vi "PC Streaming Host.vi"() -> ()   [LabVIEW 2012]
uses:
  <vilib>/userdefined/High Color/nirio_resource_hc.ctl
  <vilib>/FPGAPlugInAG/PXI-7951R/niLvFpga_Open_PXI-7951R.vi
  <vilib>/rvi/interface/common/dynamic/niFpgaDynamicAddResources.vi
  <vilib>/Utility/error.llb/Error Cluster From Error Code.vi
  <vilib>/LabVIEW Targets/FPGA/FlexRIO/CustomFPGAMethods/79XXR_Method_IOModuleStatusImpl.vi
  <vilib>/FPGAPlugInAG/Dynamic/niLvFpga_Run_Dynamic.vi
  <vilib>/rvi/errors/niLvFpgaAdjustHostInterfaceError.vi
  <vilib>/FPGAPlugInAG/Dynamic/niLvFpga_Close_Dynamic.vi
  <vilib>/rvi/interface/nirviOpenFPGA/nirviOpenFPGA.xnode
  FPGA Bitfiles/TopLevelFPGA2.0.lvbitx
  <vilib>/rvi/interface/nirviMethod/nirviMethod.xnode
  <vilib>/rvi/interface/nirviReadWriteControl/nirviReadWriteControl.xnode
  <vilib>/rvi/interface/nirviCloseFPGA/nirviCloseFPGA.xnode
  <vilib>/rvi/errors/niLvFpgaMergeErrorWithErrorCode.vi
  <vilib>/ptbypt/NI_PtbyPt.lvlib
  <vilib>/rvi/interface/Simulation/niFpgaSimulationCallBeginRW.vi
  RT_binary.vi
  NiFpgaLv.dll
  <vilib>/FPGAPlugInAG/Dynamic/niLvFpga_ConfigureFifo_Dynamic.vi
  <vilib>/FPGAPlugInAG/Dynamic/niLvFpga_StartFifo_Dynamic.vi
  <vilib>/FPGAPlugInAG/Dynamic/niLvFpga_ReadFifo_Dynamic.vi
panel:
  out "created path":path
  out "File name":string
  out "Total Data Chunks to Write":dbl
  in  "Tab Control":T1(tab)
  in  "Write mode":bool
  out "directory exists - please wait":u8(slide)
  out "directory ok":bool
  in  "Write Enable":bool
  in  "File Path":path=path "D:/Users/reuterc/Desktop"
  in  "Number of Files to Write":u32=1
  in  "Save 10% of Data?":bool
  out "File Writing Progress (%)":dbl(slide) scale=0.0..100.0
  in  "Location":i16(ring) items=["Purdue", "NIKHEF", "Zurich", "???"]
  in  "PXI address":T2 caption="RIO Device"
  in  "Trigger level":i16[](array[numeric])=[4000, 4000, 4000, 4000, 4000, 4000, 4000, 4000] caption="Trigger"
  in  "Channel 0":bool caption="Channel 1"
  in  "Channel 1":bool
  in  "Channel 2":bool caption="Channel 1"
  in  "Channel 3":bool caption="Channel 1"
  in  "Channel 4":bool caption="Channel 1"
  in  "Channel 5":bool caption="Channel 1"
  in  "Channel 6":bool caption="Channel 1"
  in  "Channel 7":bool caption="Channel 1"
  in  "Sources":string[](array[combo])
  in  "Serial numbers":string[](array[combo])
  in  "voltage":string[](array[string])
  in  "det_type":string[](array[combo])
  in  "Master Pulser On/Off":bool
  in  "Pulse duration (samples)":u32
  in  "Pulse Separation (samples)":u32
  in  "Testpulse Turnaround Time (samples)":u32=14
  in  "circular buffer length (samples)":u32=1000
  in  "Pretrigger Samples":u32=15
  out "Samples per Data Chunk":u32
  in  "Waveforms per Data Chunk":u32=5000 format="%.2p"
  in  "Samples per Waveform":u32=95
  in  "Data Chunks per File":u32=1000
  out "Average Throughput":dbl(graph)
  out "Loop Time":u32
  out "Inst. Throughput":dbl format="%#_6p"
  out "Elements in FIFO":u32(graph)
  out "FIFO Overflow":bool
  out "Current Chunk":u32
  out "Current File":i32
  out "Trigger rate":dbl(graph)
  out "Waveform Graph":dynamicdata(graph)
  out "Channel number displayed":i16=-1
  out "XML String":string
  out "error out":errorcluster
  out "UTC format?":bool=TRUE
  out "Stopped":bool
  out "Channel On/Off":bool[](array[boolean])
  in  "stop 2":bool
  in  "stop":bool
  # "Only write every 10th chunk to disk"
  # "Program will stop when number of Files to Write is Complete OR if stop is pressed."
  # "Write continuously"
  # "Write finite number of files"
  # "TODO: Make this look like the \"detectors\" tab"
  # "Waveform/Data Chunk information"
  # "To compare directly on a scope: Horizontal scale: 200 ns/div Vertical scale: ~100 mV/div If 15 pretriggers, delay = 700 ns"
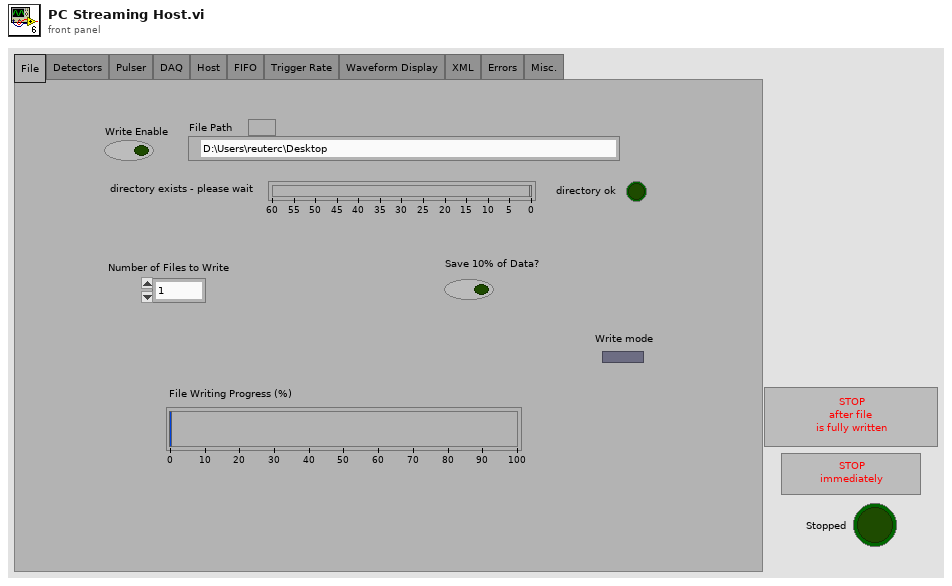
[diagram p1: front panel]
types:
  T1 = enum32{"File", "Detectors", "Pulser", "DAQ", "Host", "FIFO", "Trigger Rate", "Waveform Display", "XML", "Errors", "Misc."}
  T2 = typedef "nirio_resource_hc.ctl" = tag
  T3 = enum16{"open", "replace", "create", "open or create", "replace or create", "replace or create with confirmation"}
  T4 = enum16{"big-endian, network order", "native, host order", "little-endian"}
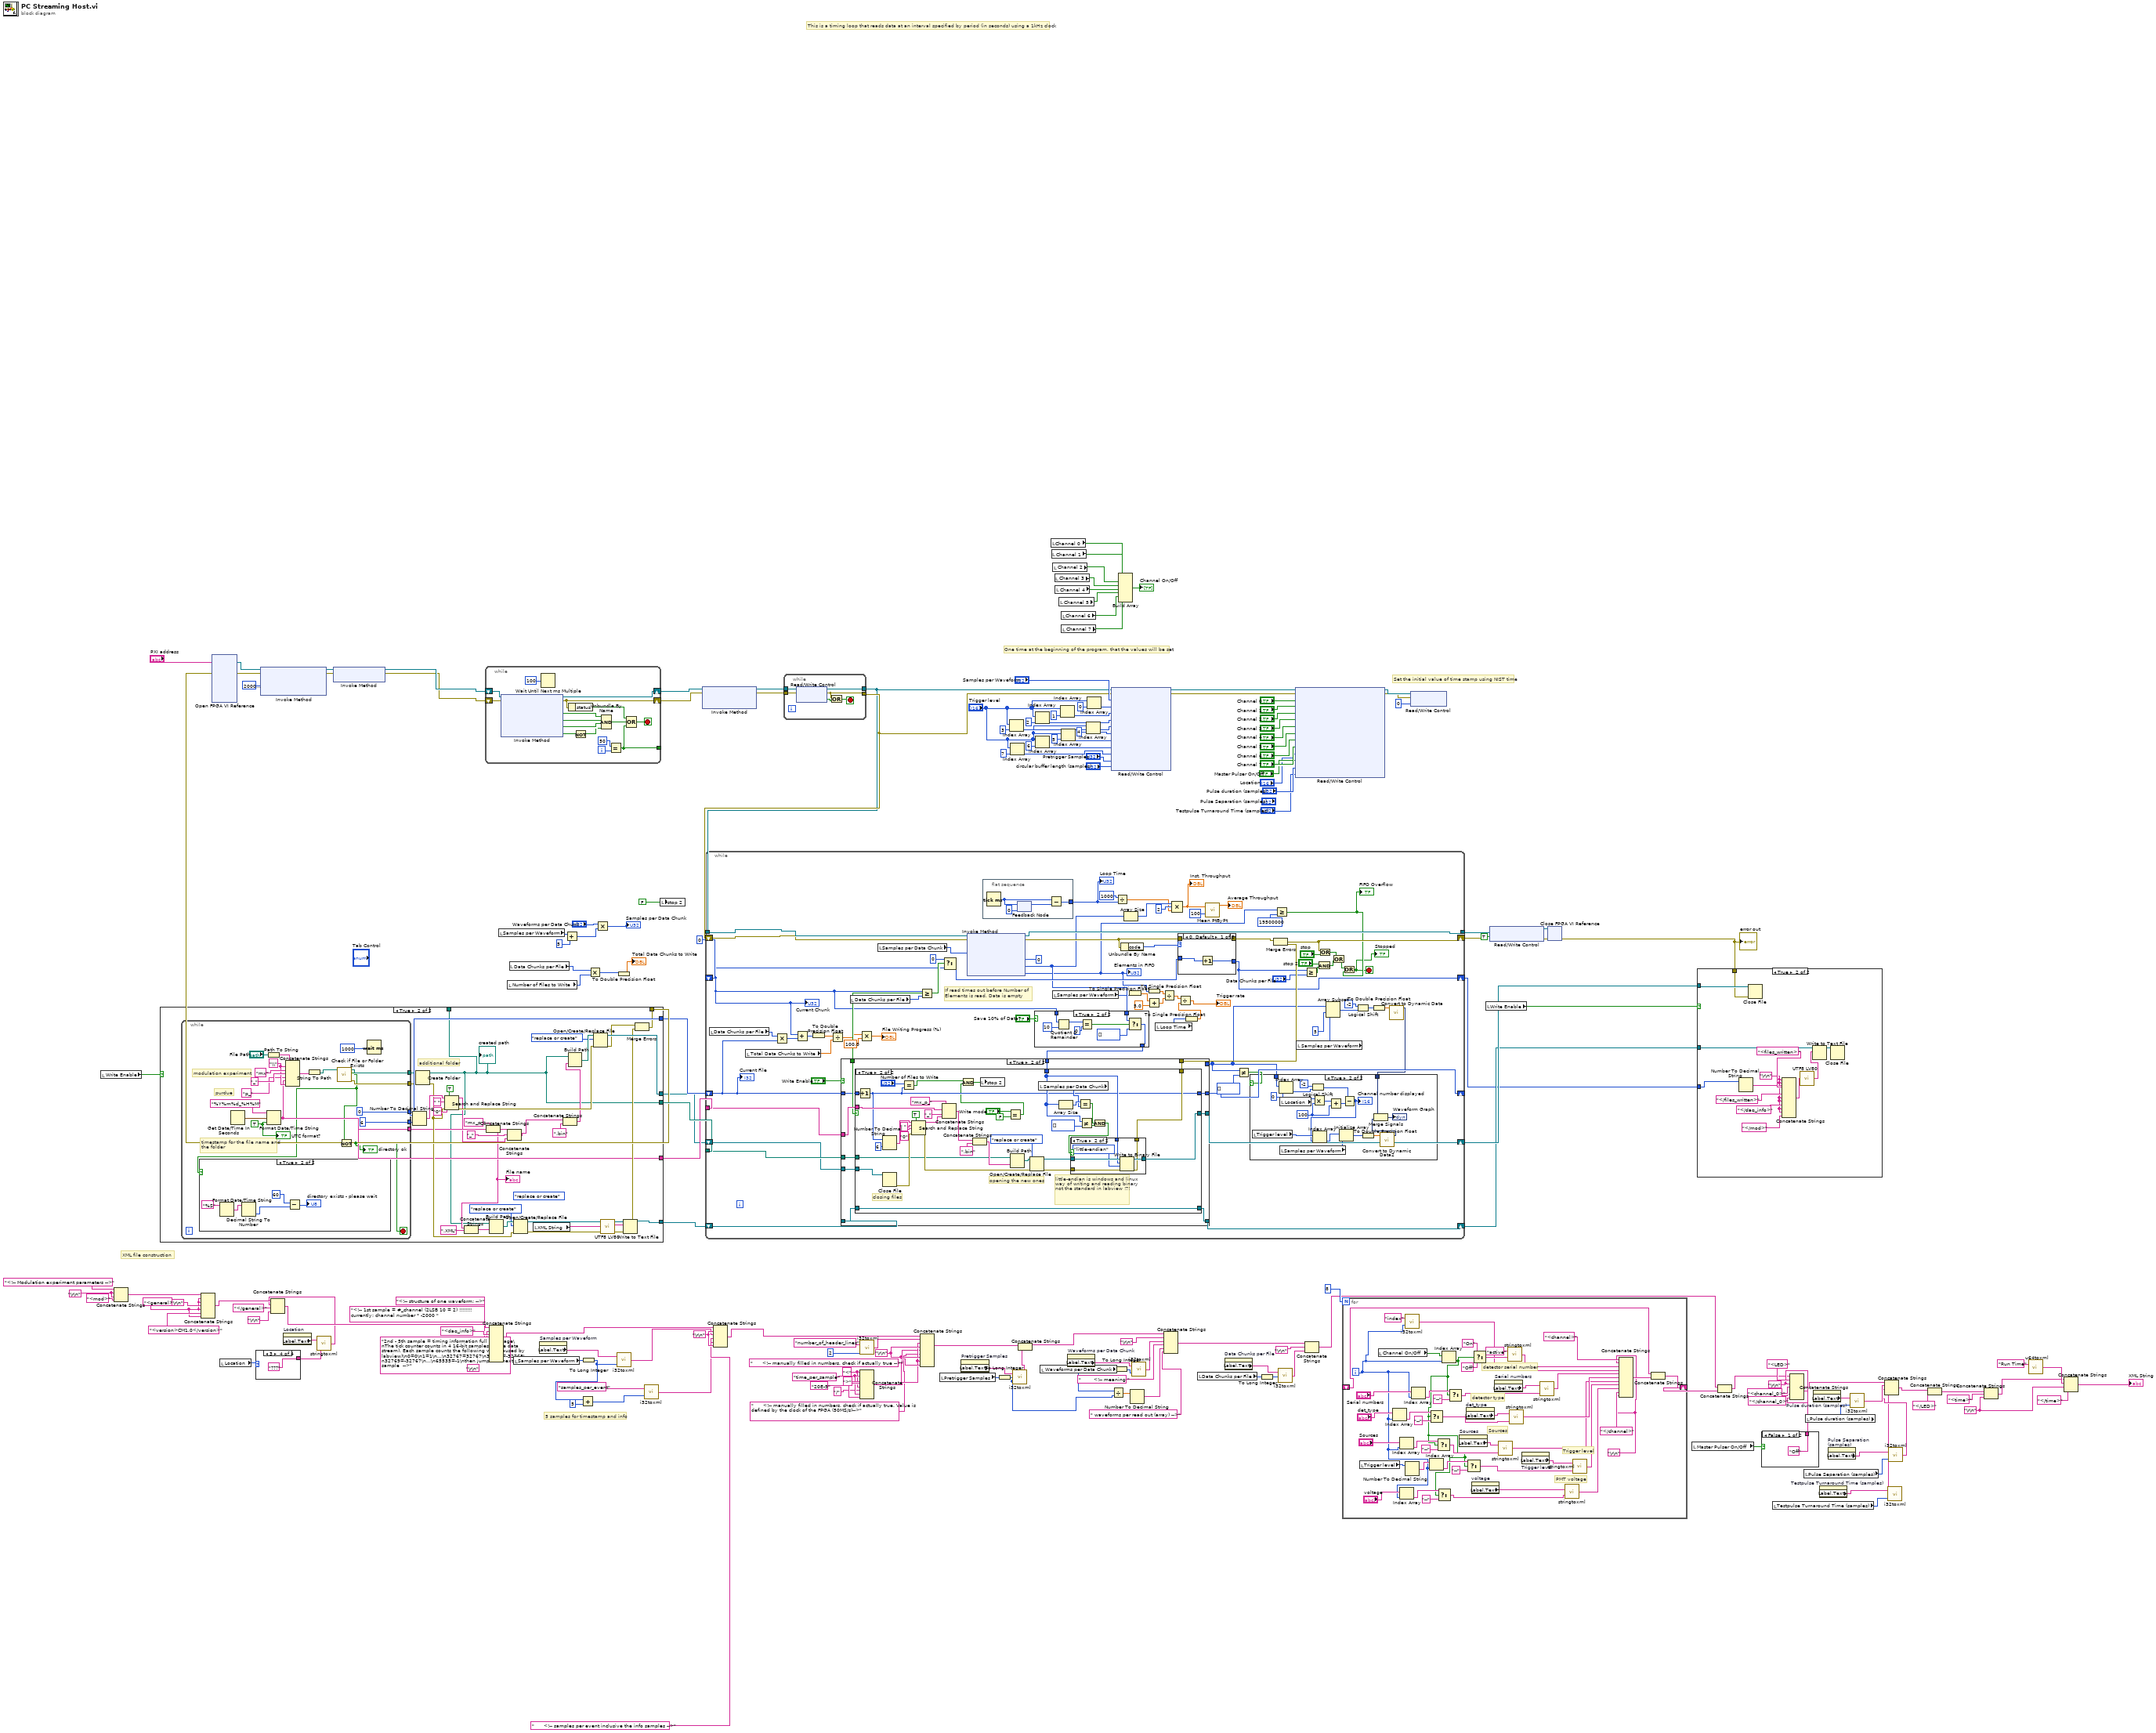
[diagram p0: block diagram]
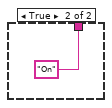
[diagram p2: hidden frame]
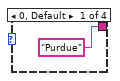
[diagram p3: hidden frame]
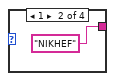
[diagram p4: hidden frame]
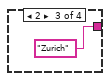
[diagram p5: hidden frame]
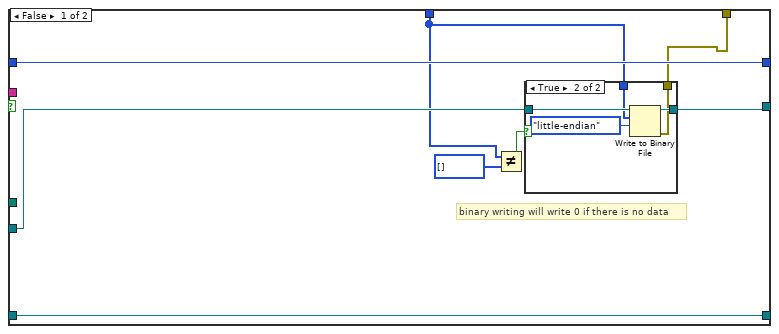
[diagram p12: hidden frame]
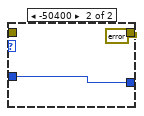
[diagram p15: hidden frame]
diagram:
  w20 = "\r\n"
  w53 = "\r\n"
  w102 = ">" ("string")
  w99 = "<" ("string")
  w101 = "time_per_sample" ("variable name")
  w106 = "      <!-- manually filled in numbers, check if actually true -->" ("string")
  w107 = "\r\n"
  w116 = "\r\n"
  w61 = "\r\n"
  w69 = "\r\n"
  w133 = "\r\n"
  # "This is a timing loop that reads data at an interval specified by period (in seconds) using a 1kHz clock"
  # "Set the initial value of time stamp using NIST time"
  # "5 samples for timestamp and info"
  # "XML file construction"
  # "One time at the beginning of the program, that the values will be set"
  n1 = local read "Write Enable"() -> (w170:bool)
  n2 = Concatenate Strings("<!-- Modulation experiment parameters -->", w133, w133, "<mod>" ("string")) -> (w73:string)
  n3 = case shown="True" w170 {
    tunnel: [_ w184] -> w175
    tunnel: [_ w193] -> w174
    tunnel: [_ w205] -> w173
    tunnel: [_ w211] -> w171
    tunnel: [_ w207] -> w169
    tunnel: [_ w194] -> w167
    tunnel: [_ w184] -> _
    frame False {
    }
    frame True {
      (unwired) T3."replace or create" ("operation (0:open)")
      # "additional folder"
      n4 = while {
        tunnel: [i16 6 ("width (-)")] -> w216
        tunnel: [0 ("number")] -> w211
        tunnel: [w225] -> w193
        tunnel: [w222] -> w187
        tunnel: [w221] -> w186
        stop <- w218 stop-if-true
        w226 = "\\" ("string")
        w230 = TRUE ("UTC format")
        # "modulation experiment"
        # "purdue"
        # "timestamp for the file name and the folder"
        n5 = Get Date/Time In Seconds() -> (seconds since 1Jan1904=w231:timestamp)
        n6 = Path To String(path="File Path") -> (string=w233:string)
        n7 = Format Date/Time String(time format string (%c)="%Y%m%d_%H%M", seconds (now)=w231, UTC format=w230) -> (date/time string=w225:string)
        n8 = Concatenate Strings(w233, w226, "mx" ("string"), "_" ("string"), "p_" ("string"), w225, w226) -> (w236:string)
        n9 = String To Path(string=w236) -> (path=w223:path)
        n10 = call <vilib>:"Check if File or Folder Exists.vi"("path"=w223) -> ("error out"=w222:errorcluster, "file or folder exists?"=w220:bool, "dup path"=w221:path)  [unwired: 8 in]
        n11 = case shown="True" w220 {
          frame False {
          }
          frame True {
            n12 = Format Date/Time String(time format string (%c)="%S") -> (date/time string=w240:string)  [unwired: 2 in]
            n13 = Decimal String To Number(string=w240) -> (number=w238:i32)  [unwired: 2 in, 1 out]
            n14 = Subtract(x=60, y=w238) -> (x-y=→"directory exists - please wait":i32)
          }
        }
        n15 = Not(x=w220) -> (.not. x?=w218:bool)
        "directory ok" <- w218
        n16 = Wait (ms)(milliseconds to wait=1000) -> ()  [unwired: 1 out]
        "UTC format?" <- w230
      }
      n17 = Number To Decimal String(number=w211, width (-)=w216) -> (decimal integer string=w215:string)
      n18 = Create Folder(path (use dialog)=w186, error in=w187) -> (created path=w184:path, error out=w202:errorcluster)  [unwired: 1 in, 1 out]
      "created path" <- w184
      n19 = Search and Replace String(replace all?=TRUE ("replace all? (F)"), input string=w215, search string=" ", replace string="0" ("replace string (\"\")"), error in=w202) -> (result string=w192:string, error out=w209:errorcluster)  [unwired: 3 in, 2 out]
      n20 = Concatenate Strings("mx_p_" ("string"), w193) -> (w185:string)
      "File name" <- w185
      n21 = Concatenate Strings(w185, ".XML" ("substring (\"\")")) -> (w199:string)
      n22 = Build Path(base path=w184, name or relative path=w199) -> (appended path=w204:path)
      n23 = Concatenate Strings(w185, "_" ("string"), w192) -> (w188:string)
      n24 = Open/Create/Replace File(file path (use dialog)=w204, error in=w202, operation (0:open)=T3."replace or create") -> (refnum out=w195:refnum<file>, error out=w197:errorcluster)  [unwired: 3 in, 1 out]
      n25 = local read "XML String"() -> (w189:string)
      n26 = Concatenate Strings(w188, ".bin" ("substring (\"\")")) -> (w201:string)
      n27 = Build Path(base path=w184, name or relative path=w201) -> (appended path=w210:path)
      n28 = Open/Create/Replace File(file path (use dialog)=w210, error in=w209, operation (0:open)=T3."replace or create") -> (refnum out=w207:refnum<file>, error out=w206:errorcluster)  [unwired: 3 in, 1 out]
      n29 = call "UTF8 LV80.vi"("text"=w189) -> ("utf-8 text out"=w190:string)
      n30 = Write to Text File(file (use dialog)=w195, text=w190, error in=w197) -> (refnum out=w194:refnum<file>, error out=w196:errorcluster)  [unwired: 1 in, 1 out]
      n31 = Merge Errors(w206, w196) -> (w205:errorcluster)
    }
  }
  n32 = Concatenate Strings(w73, w69, w69, "<general>" ("string"), w69, "<version>CM1.0</version>" ("string"), w69) -> (w74:string)
  n33 = xnode "Open FPGA VI Reference"("error in"=w173, "resource name"="PXI address") -> ("FPGA VI Reference Out"=w183:refnum<k20>, "error out"=w182:errorcluster)
  n34 = local read "Location"() -> (w71:i16)
  n35 = case shown="3" w71 {
    tunnel: ["Purdue" "NIKHEF" "Zurich" "???"] -> w70
    frame 0, Default {
    }
    frame 1 {
    }
    frame 2 {
    }
    frame 3 {
    }
  }
  n36 = xnode "Invoke Method"("FPGA VI Reference In"=w183, "error in"=w182, "Requested Depth"=u32 20000000) -> ("FPGA VI Reference Out"=w60:refnum<k20>, "error out"=w59:errorcluster)  [unwired: 1 out]
  n37 = property on="Location" class="Ring (strict)"() -> ("Label.Text"=w38:string)  [unwired: 2 in, 2 out]
  n38 = call "stringtoxml.vi"("String to write"=w70, "XML Tag"=w38) -> ("xml string"=w68:string)
  n39 = Concatenate Strings(w74, w68, "</general>" ("string"), "\r\n") -> (w75:string)
  n40 = xnode "Invoke Method"("FPGA VI Reference In"=w60, "error in"=w59) -> ("FPGA VI Reference Out"=w3:refnum<k20>, "error out"=w2:errorcluster)
  n41 = while {
    shift-right: [w252] -> w179
    shift-left: w2 -> [w260]
    shift-right: [w259] -> w12
    shift-left: w3 -> [w261]
    tunnel: [w248] -> _
    i -> [w254]
    stop <- w249 stop-if-true
    n42 = xnode "Invoke Method"("FPGA VI Reference In"=w261, "error in"=w260) -> ("FPGA VI Reference Out"=w259:refnum<k20>, "error out"=w252:errorcluster, "IO Module Present?"=w258:bool, "Power Enabled?"=w257:bool, "IO Enabled?"=w256:bool, "IO Module Mismatch?"=w247:bool)
    n43 = Wait Until Next ms Multiple(millisecond multiple=u32 100) -> ()  [unwired: 1 out]
    n44 = Unbundle By Name(w252) -> ("status"=w251:bool)
    n45 = Not(x=w247) -> (.not. x?=w246:bool)
    n46 = Compound Arithmetic op=AND(w258, w257, w256, w246) -> (w250:bool)
    n47 = Equal?(x=50, y=w254) -> (x = y?=w248:bool)
    n48 = Compound Arithmetic op=OR(w251, w250, w248) -> (w249:bool)
  }
  n49 = Concatenate Strings(w75, w61, "<daq_info>" ("string"), w61, "<!-- structure of one waveform: -->", w61, "<!-- 1st sample = #_channel (2LSB 10 = 2) !!!!!!!! currently: channel number * -2000 " ("string"), w61, "2nd - 5th sample = timing information full I16 usage\nThe tick counter counts in 4 16-bit samples (in the data stream). Each sample counts the following way (caused by labview)\n0=0\n1=1\n…\n32767=32767\n32768=-32768\n32769=-32767\n…\n65535=-1\nthen jump into next sample  -->" ("string"), w61) -> (w76:string)
  n50 = local read "Samples per Waveform"() -> (w39:u32)
  n51 = local read "Number of Files to Write"() -> (w27:u32)
  n52 = local read "Data Chunks per File"() -> (w28:u32)
  n53 = local read "Samples per Waveform"() -> (w108:u32)
  n54 = property on="Samples per Waveform" class="DigNum (strict)"() -> ("Label.Text"=w37:string)  [unwired: 2 in, 2 out]
  n55 = Add(x=w39, y=u32 5) -> (x+y=w41:u32)
  n56 = To Long Integer(number=w108) -> (32bit integer=w111:i32)
  n57 = Add(x=w111, y=5) -> (x+y=w113:i32)
  n58 = Multiply(x=w28, y=w27) -> (x*y=w26:u32)
  n59 = Multiply(x="Waveforms per Data Chunk", y=w41) -> (x*y=→"Samples per Data Chunk":u32)
  n60 = call "i32toxml.vi"("variable"=w111, "variable name"=w37) -> ("xml string"=w109:string)
  n61 = To Double Precision Float(number=w26) -> (double precision float=→"Total Data Chunks to Write":dbl)
  n62 = call "i32toxml.vi"("variable"=w113, "variable name"="samples_per_event") -> ("xml string"=w114:string)
  n63 = local write "stop 2"(FALSE ("stop 2")) -> ()
  n64 = xnode "Invoke Method"("FPGA VI Reference In"=w12, "error in"=w179) -> ("FPGA VI Reference Out"=w180:refnum<k20>, "error out"=w181:errorcluster)  [unwired: 1 in]
  n65 = Concatenate Strings(w76, w116, w109, w114, "      <!-- samples per event inclusive the info samples -->" ("string"), w116) -> (w77:string)
  n66 = while {
    tunnel: [w262] -> w135
    tunnel: [w267] -> w11
    tunnel: w180 -> [w266]
    tunnel: w181 -> [w265]
    stop <- w263 stop-if-true
    n67 = xnode "Read/Write Control"("FPGA VI Reference In"=w266, "error in"=w265) -> ("FPGA VI Reference Out"=w267:refnum<k20>, "error out"=w262:errorcluster, "Init Done"=w264:bool)
    n68 = Or(x=w262, y=w264) -> (x .or. y?=w263:bool)
  }
  n69 = while {
    shift-right: [w322] -> w14
    shift-left: w135 -> [w283]
    tunnel: w174 -> [w328]
    shift-right: [w313] -> w136
    shift-left: u32 0 -> [w291]
    tunnel: w175 -> [w329]
    shift-right: [w324] -> _
    shift-left: w171 -> [w294]
    shift-right: [w319] -> w168
    shift-left: w169 -> [w320]
    shift-right: [w316] -> w166
    shift-left: w167 -> [w317]
    tunnel: w11 -> [w284]
    tunnel: [w341] -> w15
    stop <- w268 stop-if-true
    # "If read times out before Number of Elements is read, Data is empty"
    n70 = local read "Data Chunks per File"() -> (w293:u32)
    n71 = local read "Total Data Chunks to Write"() -> (w288:dbl)
    n72 = Multiply(x=w293, y=w294) -> (x*y=w292:u32)
    n73 = Add(x=w291, y=w292) -> (x+y=w290:u32)
    n74 = To Double Precision Float(number=w290) -> (double precision float=w289:dbl)
    n75 = Divide(x=w289, y=w288) -> (x/y=w286:dbl)
    n76 = local read "Data Chunks per File"() -> (w303:u32)
    n77 = Multiply(x=w286, y=100.0) -> (x*y=→"File Writing Progress (%)":dbl)
    n78 = local read "Samples per Data Chunk"() -> (w295:u32)
    n79 = Greater Or Equal?(x=w291, y=w303) -> (x >= y?=w325:bool)
    n80 = Select(t=u32 0, s=w325, f=w291) -> (s? t:f=w326:u32)
    n81 = xnode "Invoke Method"("FPGA VI Reference In"=w284, "error in"=w283, "Number of Elements"=w295, "Timeout (ms)"=0) -> ("FPGA VI Reference Out"=w341:refnum<k20>, "error out"=w338:errorcluster, "Data"=w300:i16[], "Elements Remaining"=w282:u32)
    "Elements in FIFO" <- w282
    n82 = flat-sequence {
      tunnel: [w372] -> w332
      frame #0 {
        n83 = Tick Count (ms)() -> (millisecond timer value=w371:u32)
        n84 = feedback #1(u32 0 ("millisecond timer value")) -> (w370:u32)
        n85 = feedback-in #1(w371) -> ()
        n86 = Subtract(x=w371, y=w370) -> (x-y=w372:u32)
      }
    }
    n87 = case shown="True" "Save 10% of Data?" {
      tunnel: [w360 w363] -> w299
      tunnel: w300 -> [w360 w362]
      tunnel: w291 -> [_ w361]
      frame False {
      }
      frame True {
        n88 = Quotient & Remainder(x=w361, y=u32 10) -> (x-y*floor(x/y)=w367:u32)  [unwired: 1 out]
        n89 = Equal?(x=w367, y=u32 0) -> (x = y?=w365:bool)
        n90 = Select(t=w362, s=w365, f=i16[] [] ("y")) -> (s? t:f=w363:i16[])
      }
    }
    n91 = case shown="True" "Write Enable" {
      tunnel: w299 -> [w374 w379]
      tunnel: [w374 _] -> w296
      tunnel: w329 -> [_ w387]
      tunnel: w328 -> [_ w386]
      tunnel: w325 -> [_ w385]
      tunnel: w294 -> [w376 w384]
      tunnel: [w376 w383] -> w324
      tunnel: [_ w382] -> w321
      tunnel: [w375 w381] -> w319
      tunnel: w320 -> [w375 w380]
      tunnel: w317 -> [w373 w378]
      tunnel: [w373 w377] -> w316
      frame False {
      }
      frame True {
        n92 = case shown="True" w385 {
          tunnel: w387 -> [_ w416]
          tunnel: w386 -> [_ w423]
          tunnel: w379 -> [w389 w413]
          tunnel: [w388 w415] -> w382
          tunnel: w380 -> [w394 w431]
          tunnel: w384 -> [w395 w432]
          tunnel: [w395 w407] -> w383
          tunnel: [w393 w424] -> w381
          tunnel: w378 -> [w392 w418]
          tunnel: [w392 w418] -> w377
          frame False {
            # "binary writing will write 0 if there is no data"
            n93 = Not Equal?(x=w389, y=i16[] []) -> (x != y?=w390:bool)
            n94 = case shown="True" w390 {
              tunnel: w394 -> [w396 w401]
              tunnel: [w396 w400] -> w393
              tunnel: [_ w399] -> w388
              tunnel: w389 -> [_ w397]
              frame False {
              }
              frame True {
                n95 = Write to Binary File(file (use dialog)=w401, data=w397, 9:T4."little-endian" ("byte order (0:big-endian, network order)")) -> (refnum out=w400:refnum<file>, error out=w399:errorcluster)  [unwired: 3 in, 1 out]
              }
            }
          }
          frame True {
            # "opening the new ones"
            # "closing files"
            # "little-endian is windows and linux way of writing and reading binary not the standard in labview !?!"
            n96 = Increment(x=w432) -> (x+1=w407:i32)
            n97 = Number To Decimal String(number=w407, width (-)=i16 6) -> (decimal integer string=w434:string)
            n98 = Close File(refnum=w431) -> (error out=w430:errorcluster)  [unwired: 1 in, 1 out]
            n99 = Equal?(x="Number of Files to Write", y=w407) -> (x = y?=w402:bool)
            n100 = Search and Replace String(replace all?=TRUE ("replace all? (F)"), input string=w434, search string=" ", replace string="0" ("replace string (\"\")"), error in=w430) -> (result string=w422:string, error out=w429:errorcluster)  [unwired: 3 in, 2 out]
            n101 = Concatenate Strings("mx_p_" ("string"), w423, "_" ("string"), w422) -> (w417:string)
            n102 = Concatenate Strings(w417, ".bin" ("substring (\"\")")) -> (w420:string)
            n103 = Equal?(x="Write mode", y=FALSE) -> (x = y?=w403:bool)
            n104 = And(x=w402, y=w403) -> (x .and. y?=w404:bool)
            n105 = local write "stop 2"(w404) -> ()
            n106 = Build Path(base path=w416, name or relative path=w420) -> (appended path=w428:path)
            n107 = Open/Create/Replace File(file path (use dialog)=w428, error in=w429, operation (0:open)=T3."replace or create") -> (refnum out=w425:refnum<file>, error out=w426:errorcluster)  [unwired: 3 in, 1 out]
            n108 = local read "Samples per Data Chunk"() -> (w411:u32)
            n109 = Array Size(array=w413) -> (size(s)=w412:i32)
            n110 = Equal?(x=w412, y=w411) -> (x = y?=w410:bool)
            n111 = Not Equal?(x=w413, y=i16[] []) -> (x != y?=w414:bool)
            n112 = And(x=w414, y=w410) -> (x .and. y?=w409:bool)
            n113 = case shown="True" w409 {
              tunnel: w426 -> [w440 w447]
              tunnel: w425 -> [w441 w446]
              tunnel: [w441 w445] -> w424
              tunnel: [w440 w444] -> w415
              tunnel: w413 -> [_ w443]
              frame False {
              }
              frame True {
                n114 = Write to Binary File(file (use dialog)=w446, data=w443, error in=w447, 9:T4."little-endian" ("byte order (0:big-endian, network order)")) -> (refnum out=w445:refnum<file>, error out=w444:errorcluster)  [unwired: 2 in, 1 out]
              }
            }
          }
        }
      }
    }
    n115 = local read "Samples per Waveform"() -> (w278:u32)
    n116 = Divide(x=u32 1000, y=w332) -> (x/y=w334:dbl)
    n117 = Unbundle By Name(w338) -> ("code"=w339:i32)
    n118 = Array Size(array=w300) -> (size(s)=w337:i32)
    n119 = To Single Precision Float(number=w278) -> (single precision float=w277:sgl)
    n120 = To Single Precision Float(number=w282) -> (single precision float=w281:sgl)
    n121 = Add(x=w277, y=5.0) -> (x+y=w280:dbl)
    n122 = local read "Loop Time"() -> (w275:u32)
    n123 = Divide(x=w281, y=w280) -> (x/y=w276:dbl)
    n124 = Compound Arithmetic op=MULTIPLY(w337, 2 ("y"), w334) -> (w331:dbl)
    "Inst. Throughput" <- w331
    n125 = case shown="0, Default" w339 {
      tunnel: [w450 errorcluster {"status"=FALSE, "code"=0, "source"=""} ("error constant")] -> w323
      tunnel: w338 -> [w450 _]
      tunnel: w326 -> [w449 w451]
      tunnel: [w448 w451] -> w313
      frame 0, Default {
        n126 = Increment(x=w449) -> (x+1=w448:u32)
      }
      frame -50400 {
      }
    }
    n127 = To Single Precision Float(number=w275) -> (single precision float=w274:sgl)
    n128 = Divide(x=w276, y=w274) -> (x/y=→"Trigger rate":dbl)
    n129 = call <vilib>:"Mean PtByPt.vi"("x"=w331, "sample length"=100) -> ("mean"=→"Average Throughput":dbl)  [unwired: 2 in, 1 out]
    n130 = Not Equal?(x=w296, y=i16[] []) -> (x != y?=w297:bool)
    n131 = Merge Errors(w323, w321) -> (w322:errorcluster)
    n132 = Greater Or Equal?(x=w282, y=u32 19500000) -> (x >= y?=w304:bool)
    "FIFO Overflow" <- w304
    n133 = local read "Samples per Waveform"() -> (w306:u32)
    n134 = Greater Or Equal?(x=w313, y="Data Chunks per File") -> (x >= y?=w315:bool)
    n135 = And(x="stop 2", y=w315) -> (x .and. y?=w314:bool)
    n136 = Or(x=w322, y="stop") -> (x .or. y?=w311:bool)
    n137 = Array Subset(array=w296, index=5, length=w306) -> (w270:i16[])
    n138 = Or(x=w311, y=w314) -> (x .or. y?=w309:bool)
    n139 = Or(x=w309, y=w304) -> (x .or. y?=w268:bool)
    "Stopped" <- w268
    n140 = Logical Shift(y=i16 -2, x=w270) -> (x << y=w269:i16[])
    n141 = To Double Precision Float(number=w269) -> (double precision float=w305:dbl[])
    n142 = call "Convert to Dynamic Data"("Array"=w305) -> ("Dynamic Data Type"=w272:dynamicdata)  [unwired: 3 in]
    n143 = case shown="True" w297 {
      tunnel: w296 -> [_ w358]
      tunnel: w272 -> [_ w345]
      frame False {
      }
      frame True {
        w352 = i16 100
        n144 = local read "Trigger level"() -> (w347:i16[])
        n145 = Index Array(array=w358, index=0) -> (element=w355:i16)
        n146 = local read "Samples per Waveform"() -> (w349:u32)
        n147 = local read "Location"() -> (w351:i16)
        n148 = Logical Shift(y=i16 -2, x=w355) -> (x << y=w357:i16)
        n149 = Multiply(x=w351, y=w352) -> (x*y=w353:i16)
        n150 = Add(x=w353, y=w352) -> (x+y=w354:i16)
        n151 = Subtract(x=w357, y=w354) -> (x-y=w342:i16)
        "Channel number displayed" <- w342
        n152 = Index Array(array=w347, index=w342) -> (element=w348:i16)
        n153 = Initialize Array(w348, w349) -> (w343:i16[])
        n154 = To Double Precision Float(number=w343) -> (double precision float=w350:dbl[])
        n155 = call "Convert to Dynamic Data2"("Array"=w350) -> ("Dynamic Data Type"=w344:dynamicdata)  [unwired: 3 in]
        n156 = Merge Signals(w345, w344) -> (→"Waveform Graph":dynamicdata)
      }
    }
    "Loop Time" <- w332
    "Current Chunk" <- w291
    "Current File" <- w294
  }
  n157 = call "i32toxml.vi"("variable"=2, "variable name"="number_of_header_lines") -> ("xml string"=w96:string)
  n158 = Concatenate Strings(w99, w101, w102, "20E-9" ("string"), w99, "/" ("string"), w101, w102) -> (w104:string)
  n159 = Concatenate Strings(w77, w96, w106, w107, w104, "      <!-- manually filled in numbers, check if actually true. Value is defined by the clock of the FPGA (50MS/s)-->" ("string"), w107, w106, w107) -> (w78:string)
  n160 = local read "Pretrigger Samples"() -> (w94:u32)
  n161 = property on="Pretrigger Samples" class="DigNum (strict)"() -> ("Label.Text"=w36:string)  [unwired: 2 in, 2 out]
  n162 = To Long Integer(number=w94) -> (32bit integer=w85:i32)
  n163 = Index Array(array="Trigger level", index=3) -> (element=w157:i16)
  n164 = Index Array(array="Trigger level", index=7) -> (element=w149:i16)
  n165 = call "i32toxml.vi"("variable"=w85, "variable name"=w36) -> ("xml string"=w95:string)
  n166 = Concatenate Strings(w78, w95) -> (w79:string)
  n167 = Index Array(array="Trigger level", index=2) -> (element=w160:i16)
  n168 = Index Array(array="Trigger level", index=6) -> (element=w150:i16)
  n169 = local read "Waveforms per Data Chunk"() -> (w90:u32)
  n170 = local read "Channel 0"() -> (w126:bool)
  n171 = local read "Channel 1"() -> (w125:bool)
  n172 = local read "Channel 2"() -> (w124:bool)
  n173 = local read "Channel 3"() -> (w123:bool)
  n174 = local read "Channel 4"() -> (w122:bool)
  n175 = local read "Channel 5"() -> (w121:bool)
  n176 = Index Array(array="Trigger level", index=1) -> (element=w159:i16)
  n177 = local read "Channel 6"() -> (w120:bool)
  n178 = Index Array(array="Trigger level", index=5) -> (element=w151:i16)
  n179 = local read "Channel 7"() -> (w119:bool)
  n180 = property on="Waveforms per Data Chunk" class="DigNum (strict)"() -> ("Label.Text"=w35:string)  [unwired: 2 in, 2 out]
  n181 = Index Array(array="Trigger level", index=4) -> (element=w152:i16)
  n182 = Index Array(array="Trigger level", index=0) -> (element=w146:i16)
  n183 = xnode "Read/Write Control"("FPGA VI Reference In"=w11, "error in"=w135, "Record Size only data"="Samples per Waveform", "Trigger 0"=w146, "Trigger 1"=w159, "Trigger 2"=w160, "Trigger 3"=w157, "Trigger 4"=w152, "Trigger 5"=w151, "Trigger 6"=w150, "Trigger 7"=w149, "# of pretrigger"="Pretrigger Samples", "circular buffer length"="circular buffer length (samples)") -> ("FPGA VI Reference Out"=w148:refnum<k20>, "error out"=w147:errorcluster)
  n184 = Divide(x=w90, y=w85) -> (x/y=w89:dbl)
  n185 = To Long Integer(number=w90) -> (32bit integer=w88:i32)
  n186 = Build Array(w126, w125, w124, w123, w122, w121, w120, w119) -> (→"Channel On/Off":bool[])
  n187 = Number To Decimal String(number=w89) -> (decimal integer string=w92:string)  [unwired: 1 in]
  n188 = call "i32toxml.vi"("variable"=w88, "variable name"=w35) -> ("xml string"=w86:string)
  n189 = Concatenate Strings(w79, "\r\n", w86, "        <!-- meaning " ("string"), w92, " waveforms per read out (array) -->" ("string")) -> (w80:string)
  n190 = local read "Data Chunks per File"() -> (w83:u32)
  n191 = property on="Data Chunks per File" class="DigNum (strict)"() -> ("Label.Text"=w34:string)  [unwired: 2 in, 2 out]
  n192 = To Long Integer(number=w83) -> (32bit integer=w82:i32)
  n193 = call "i32toxml.vi"("variable"=w82, "variable name"=w34) -> ("xml string"=w81:string)
  n194 = xnode "Read/Write Control"("FPGA VI Reference In"=w148, "error in"=w147, "channel 0 on/off"="Channel 0", "channel 1 on/off"="Channel 1", "channel 2 on/off"="Channel 2", "channel 3 on/off"="Channel 3", "channel 4 on/off"="Channel 4", "channel 5 on/off"="Channel 5", "channel 6 on/off"="Channel 6", "channel 7 on/off"="Channel 7", "Location"="Location", "Testpulser On/Off"="Master Pulser On/Off", "Testpulse duration (20 ns ticks)"="Pulse duration (samples)", "Testpulse Time Delay (20 ns ticks)"="Testpulse Turnaround Time (samples)") -> ("FPGA VI Reference Out"=w10:refnum<k20>, "error out"=w9:errorcluster)
  n195 = Concatenate Strings(w80, "\r\n", w81) -> (w5:string)
  n196 = for {
    N: 8 -> [_]
    shift-right: [w456] -> w6
    shift-left: _ -> [w455]
    i -> [w463]
    w453 = "\r\n"
    # "PMT voltage"
    # "Trigger level"
    # "Sources"
    # "detector type"
    # "detector serial number"
    n197 = local read "Trigger level"() -> (w473:i16[])
    n198 = local read "Channel On/Off"() -> (w499:bool[])
    n199 = Index Array(array="det_type", index=w463) -> (element=w483:string)
    n200 = Index Array(array="Sources", index=w463) -> (element=w478:string)
    n201 = Index Array(array="voltage", index=w463) -> (element=w465:string)
    n202 = call "i32toxml.vi"("variable"=w463, "variable name"="index") -> ("xml string"=w493:string)
    n203 = Number To Decimal String(number=w473) -> (decimal integer string=w470:string[])  [unwired: 1 in]
    n204 = Index Array(array="Serial numbers", index=w463) -> (element=w490:string)
    n205 = Index Array(array=w470, index=w463) -> (element=w471:string)
    n206 = Index Array(array=w499, index=w463) -> (element=w462:bool)
    n207 = Select(t=w483, s=w462, f="--") -> (s? t:f=w481:string)
    n208 = Select(t=w478, s=w462, f="--") -> (s? t:f=w475:string)
    n209 = Select(t=w465, s=w462, f="--") -> (s? t:f=w461:string)
    n210 = Select(t=w490, s=w462, f="--") -> (s? t:f=w488:string)
    n211 = property on="Sources" class="Arr (strict)"() -> ("Label.Text"=w476:string)  [unwired: 2 in, 2 out]
    n212 = property on="det_type" class="Arr (strict)"() -> ("Label.Text"=w482:string)  [unwired: 2 in, 2 out]
    n213 = Select(t=w471, s=w462, f="--") -> (s? t:f=w469:string)
    n214 = property on="voltage" class="Arr (strict)"() -> ("Label.Text"=w460:string)  [unwired: 2 in, 2 out]
    n215 = Select(t="On" ("List Name"), s=w462, f="Off" ("List Name")) -> (s? t:f=w495:string)
    n216 = property on="Serial numbers" class="Arr (strict)"() -> ("Label.Text"=w487:string)  [unwired: 2 in, 2 out]
    n217 = call "stringtoxml.vi"("String to write"=w475, "XML Tag"=w476) -> ("xml string"=w474:string)
    n218 = call "stringtoxml.vi"("String to write"=w495, "XML Tag"="active") -> ("xml string"=w492:string)
    n219 = call "stringtoxml.vi"("String to write"=w481, "XML Tag"=w482) -> ("xml string"=w480:string)
    n220 = property on="Trigger level" class="Arr (strict)"() -> ("Label.Text"=w468:string)  [unwired: 2 in, 2 out]
    n221 = call "stringtoxml.vi"("String to write"=w488, "XML Tag"=w487) -> ("xml string"=w486:string)
    n222 = call "stringtoxml.vi"("String to write"=w461, "XML Tag"=w460) -> ("xml string"=w459:string)
    n223 = call "stringtoxml.vi"("String to write"=w469, "XML Tag"=w468) -> ("xml string"=w467:string)
    n224 = Concatenate Strings("<channel>" ("List Name"), w453, w493, w492, w486, w480, w474, w467, w459, "</channel>" ("List Name"), w453) -> (w457:string)
    n225 = Concatenate Strings(w455, w457) -> (w456:string)
  }
  n226 = xnode "Read/Write Control"("FPGA VI Reference In"=w10, "error in"=w9, "initial value"=u64 0) -> ()  [unwired: 2 out]
  n227 = local read "Write Enable"() -> (w176:bool)
  n228 = xnode "Read/Write Control"("FPGA VI Reference In"=w15, "error in"=w14, "Stop FPGA and exit"=TRUE) -> ("FPGA VI Reference Out"=w44:refnum<k20>, "error out"=w43:errorcluster)
  n229 = xnode "Close FPGA VI Reference"("FPGA VI Reference In"=w44, "error in"=w43) -> ("error out"=w177:errorcluster)
  "error out" <- w177
  n230 = local read "Master Pulser On/Off"() -> (w56:bool)
  n231 = case shown="True" w176 {
    tunnel: w177 -> [_ w503]
    tunnel: w168 -> [_ w512]
    tunnel: w166 -> [_ w511]
    tunnel: w136 -> [_ w506]
    frame False {
    }
    frame True {
      w500 = "\r\n"
      n232 = Number To Decimal String(number=w506) -> (decimal integer string=w508:string)  [unwired: 1 in]
      n233 = Close File(refnum=w512, error in=w503) -> ()  [unwired: 2 out]
      n234 = Concatenate Strings(w500, w500, "<files_written> " ("text"), w508, "</files_written>" ("string"), w500, w500, "</daq_info>" ("string"), w500, w500, "</mod>" ("string")) -> (w502:string)
      n235 = call "UTF8 LV80.vi"("text"=w502) -> ("utf-8 text out"=w504:string)
      n236 = Write to Text File(file (use dialog)=w511, text=w504) -> (refnum out=w510:refnum<file>)  [unwired: 2 in, 2 out]
      n237 = Close File(refnum=w510) -> ()  [unwired: 1 in, 2 out]
    }
  }
  n238 = Concatenate Strings(w5, w6) -> (w4:string)
  n239 = case shown="False" w56 {
    tunnel: ["Off" "On"] -> w55
    frame False {
    }
    frame True {
    }
  }
  n240 = local read "Testpulse Turnaround Time (samples)"() -> (w47:u32)
  n241 = Concatenate Strings(w4, "<LED>" ("string"), w53, "<channel_0>" ("string"), w55, "</channel_0>" ("string"), w53) -> (w51:string)
  n242 = local read "Pulse Separation (samples)"() -> (w50:u32)
  n243 = local read "Pulse duration (samples)"() -> (w52:u32)
  n244 = property on="Pulse duration (samples)" class="DigNum (strict)"() -> ("Label.Text"=w33:string)  [unwired: 2 in, 2 out]
  n245 = property on="Testpulse Turnaround Time (samples)" class="DigNum (strict)"() -> ("Label.Text"=w32:string)  [unwired: 2 in, 2 out]
  n246 = property on="Pulse Separation (samples)" class="DigNum (strict)"() -> ("Label.Text"=w31:string)  [unwired: 2 in, 2 out]
  n247 = call "i32toxml.vi"("variable"=w52, "variable name"=w33) -> ("xml string"=w49:string)
  n248 = call "i32toxml.vi"("variable"=w47, "variable name"=w32) -> ("xml string"=w46:string)
  n249 = call "i32toxml.vi"("variable"=w50, "variable name"=w31) -> ("xml string"=w48:string)
  n250 = Concatenate Strings(w51, w49, w48, w46) -> (w24:string)
  n251 = Concatenate Strings(w24, "</LED>" ("string")) -> (w23:string)
  n252 = Concatenate Strings(w23, "<time>" ("string"), w20) -> (w13:string)
  n253 = call "u64toxml.vi"("variable name"="Run Time") -> ("xml string"=w19:string)  [unwired: 1 in]
  n254 = Concatenate Strings(w13, w19, w20, "</time>" ("string")) -> (→"XML String":string)
